vi "Meas_EIS_Spectra_Polar_v6 - temp.vi"(9 "output cluster":T1, 10 "testp":T2={"Start F"=1.0, "Stop F"=10000.0, "# Steps"=50, "Init Z Guess"=1.0, "Device #"=0, "Vdrive (V)"=0.1} caption="Test Parameters" {"Vdrive (V)" min=0.0001 max=10; "Device #" min=0 max=10 step=1; "Init Z Guess" format="%_5f"; "# Steps" min=1 max=1800 step=1; "Stop F" min=0.0010000000474974513 max=2000000.0 step=0.001 format="%#_3f"; "Start F" min=0.0010000000474974513 max=2000000.0 step=0.001 format="%#_3f"}, 11 "Output file refnum":refnum<file>) -> ()   [LabVIEW 2018]
uses:
  AC States cntrl.ctl
panel:
  out "Init Z Guess":sgl
  in  "Tab Control":enum32{"Outputs", "TakeData"}(tab)
  out "XY Graph":cluster{sgl, sgl}[](graph)
  out "IERange":i32
  out "IchRange":i32
  out "VchRange":i32
  out "Index no.":i32=1
  out "Zphz":dbl
  out "Zmod":dbl
  out "Zfreq":dbl
  in  "Control Mode":i32(ring)=1 items=["GstatMode", "PstatMode", "ZRAMode", "FRAMode"]
  out "Data Available":bool
  out "Status":enum16{"Ok", "Retry", "Error", "Done"}(ring)
  out "NumPoints":i32
  in  "Freqin":sgl=1000.0 format="%#_3g"
  out "event callback refnum":refnum<k27>
  out "Section":string
  out "ReadZ":refnum<k7>
  out "Pstat":refnum<k7>
  out "Device List":refnum<k7>
  out "Data Acquisition Complete":bool
  in  "GAMRYCOMLib.IGamryReadZ":refnum<k7>
  in  "GAMRYCOMLib.IGamryPstat":refnum<k7>
  in  "GAMRYCOMLib.IGamryDeviceList":refnum<k7>
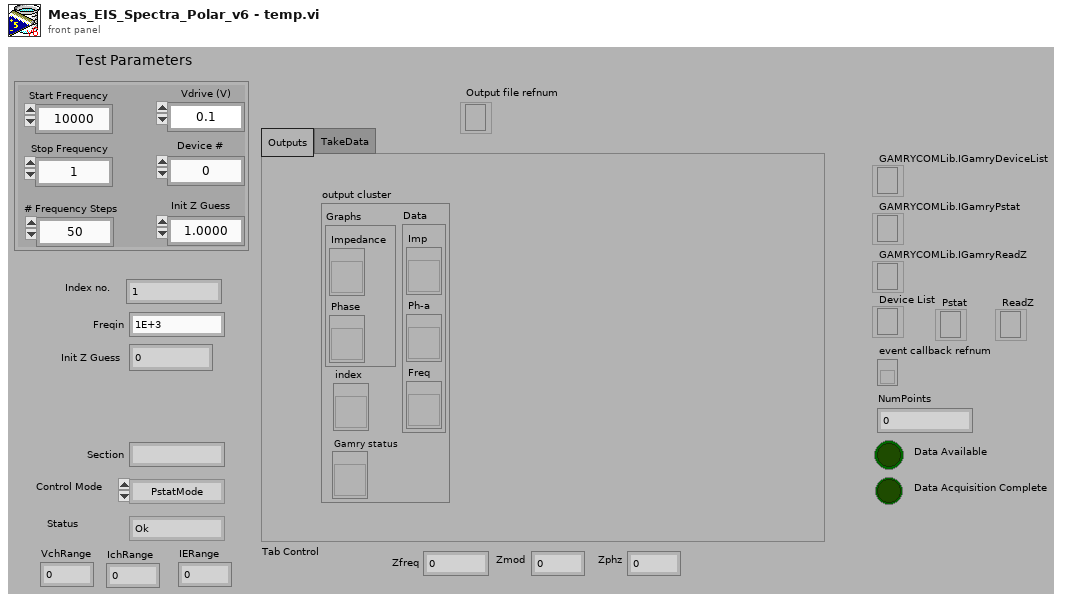
[diagram p1: front panel]
types:
  T1 = cluster{"Data":cluster{"Imp":refnum<vi>, "Ph-a":refnum<vi>, "Freq":refnum<vi>}, "Graphs":cluster{"Impedance":refnum<vi>, "Phase":refnum<vi>}, "index":refnum<vi>, "Gamry status":refnum<vi>}
  T2 = cluster{"Start F":dbl, "Stop F":dbl, "# Steps":u32, "Init Z Guess":sgl, "Device #":i16, "Vdrive (V)":sgl}
  T3 = typedef "AC States cntrl.ctl" = enum16{"Initialize Variables", "Initialize Pstat", "Initialize Dtaq", "Settings", "Frequency calc", "Set Cycle Limits", "Take Data", "Read Z Measure", "Cleanup", "Stop"}
  T4 = cluster{"Imp":refnum<vi>, "Ph-a":refnum<vi>, "Freq":refnum<vi>}
  T5 = cluster{"Impedance":refnum<vi>, "Phase":refnum<vi>}
  T6 = cluster{"Data Acquisition Complete":refnum<vi>, "Status":refnum<vi>}
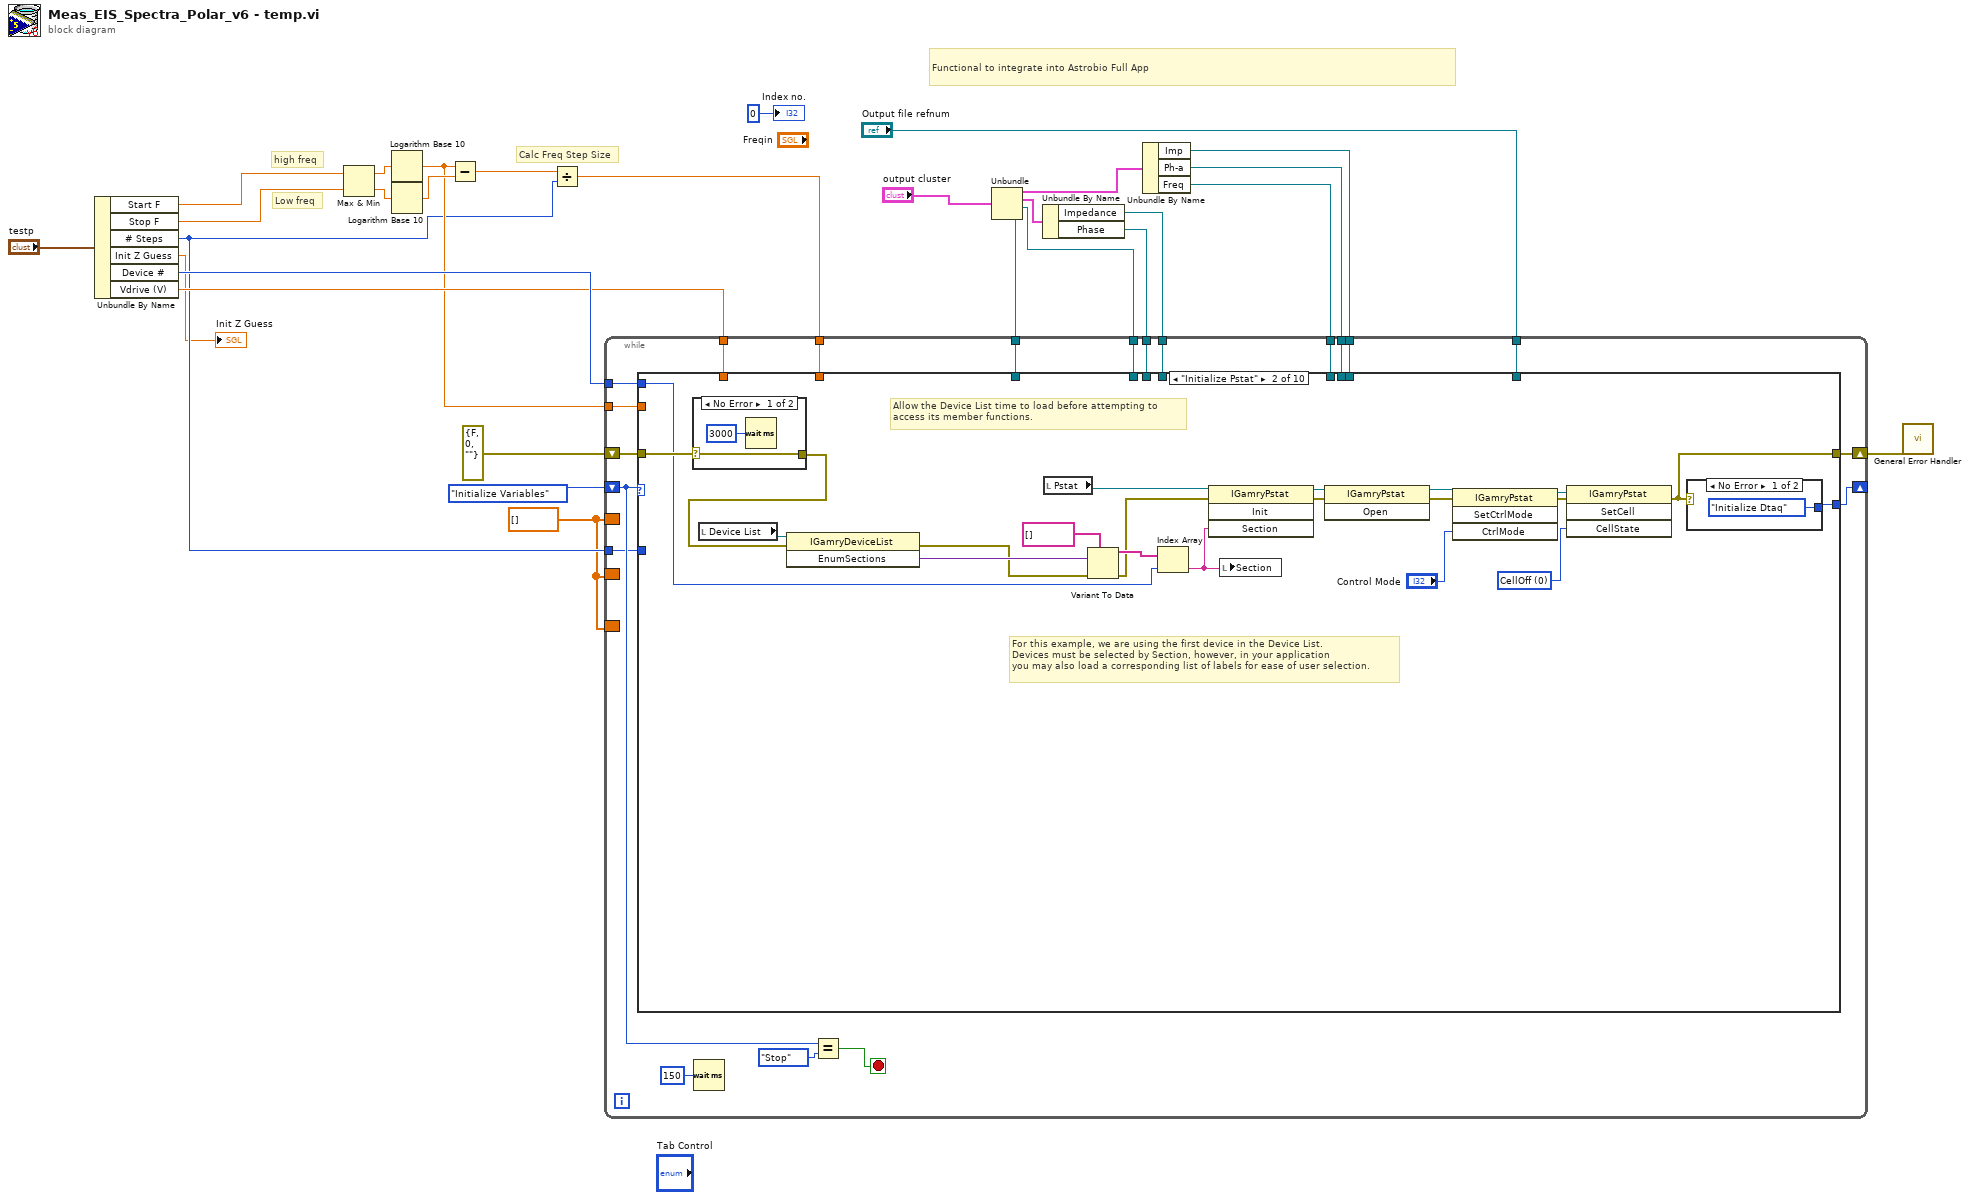
[diagram p0: block diagram]
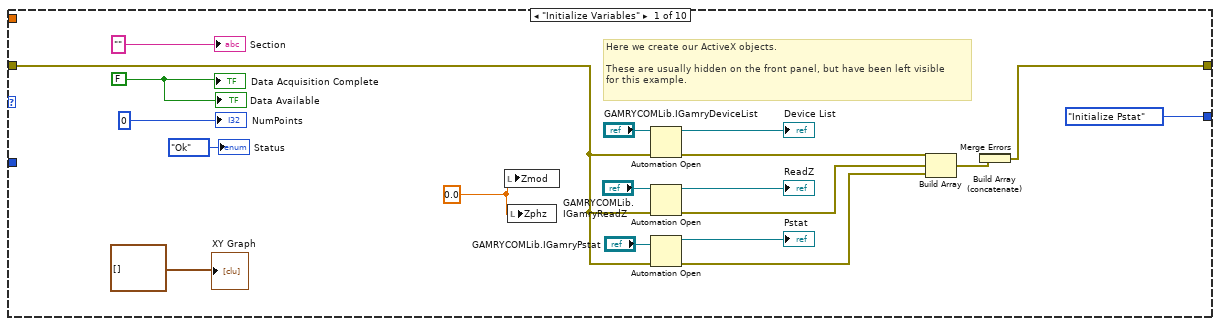
[diagram p2: hidden frame]
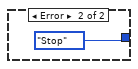
[diagram p4: hidden frame]
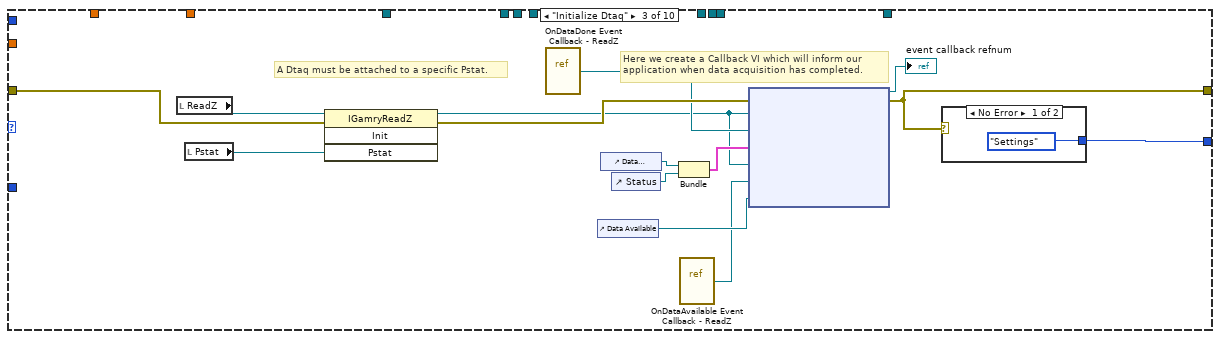
[diagram p5: hidden frame]
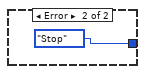
[diagram p6: hidden frame]
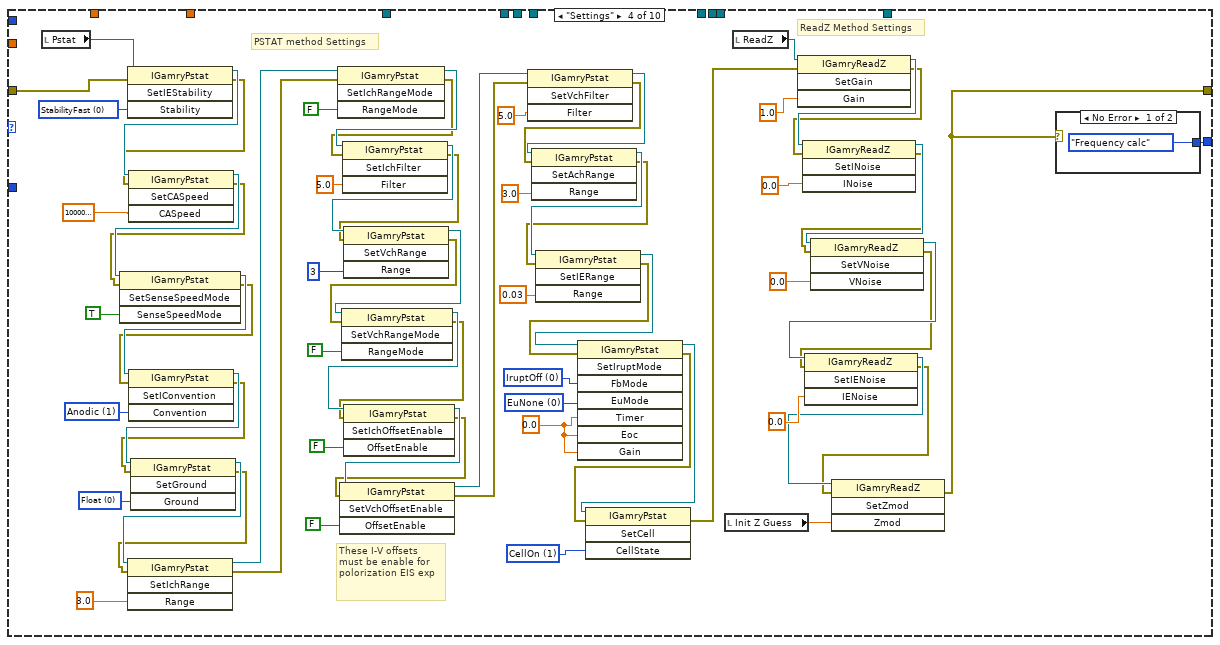
[diagram p7: hidden frame]
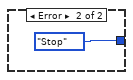
[diagram p8: hidden frame]
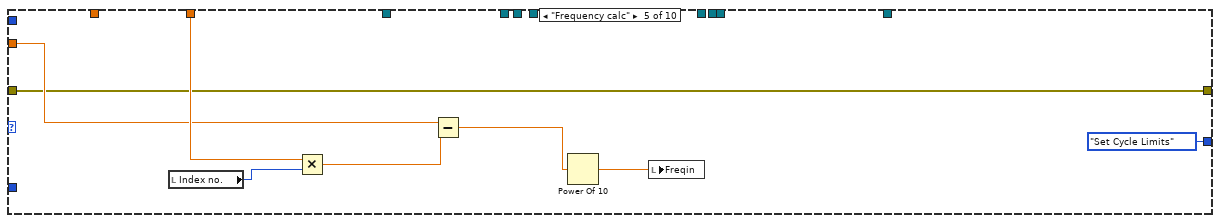
[diagram p9: hidden frame]
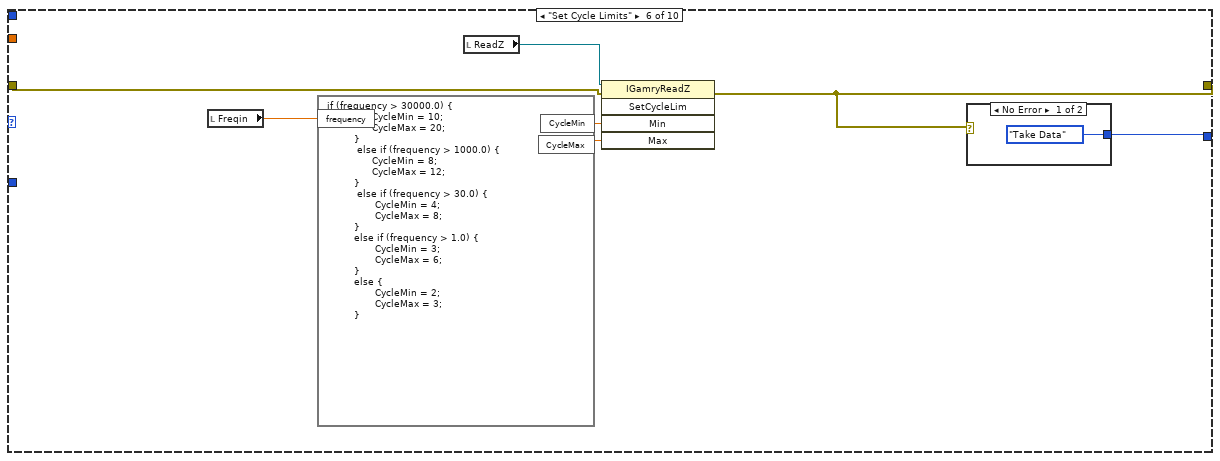
[diagram p10: hidden frame]
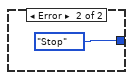
[diagram p11: hidden frame]
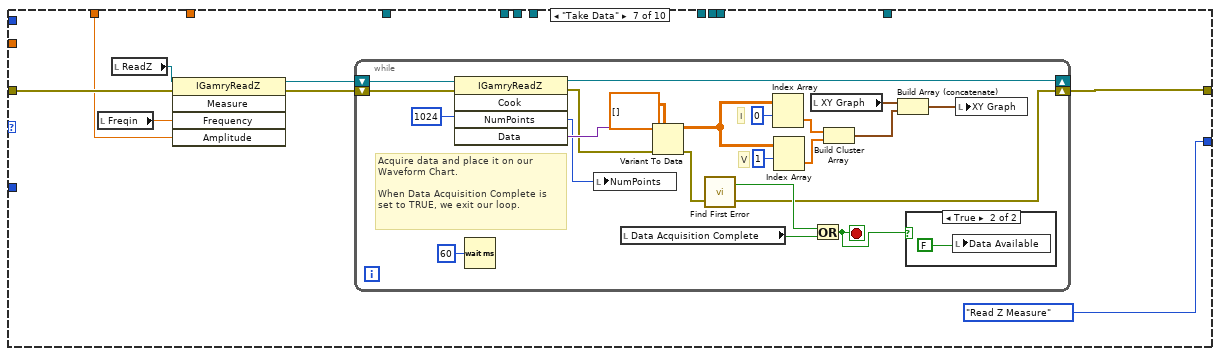
[diagram p12: hidden frame]
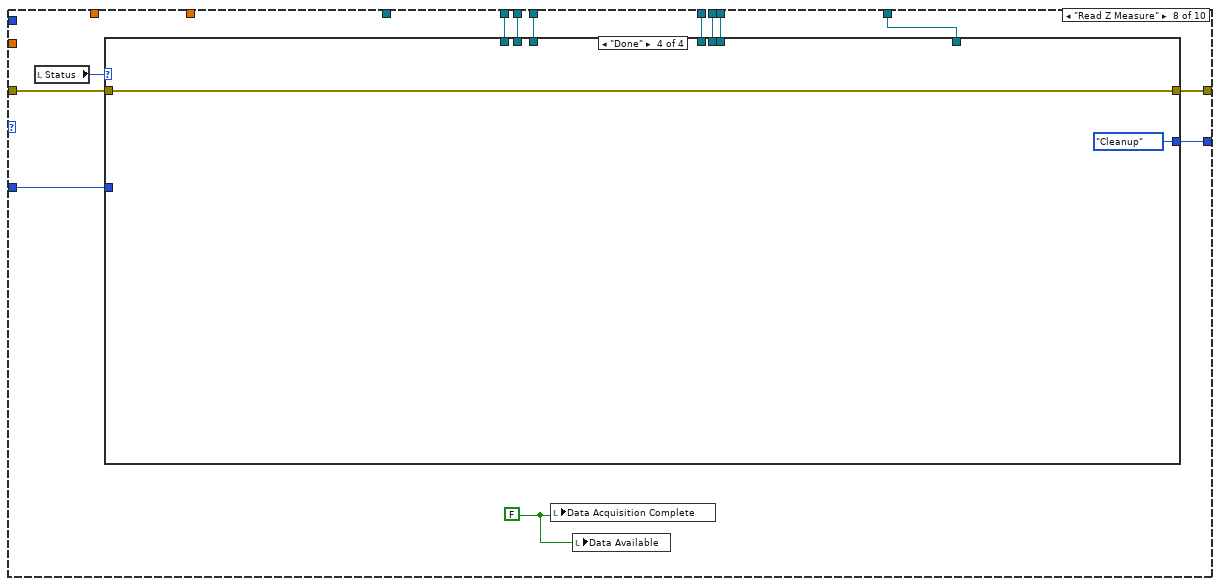
[diagram p14: hidden frame]
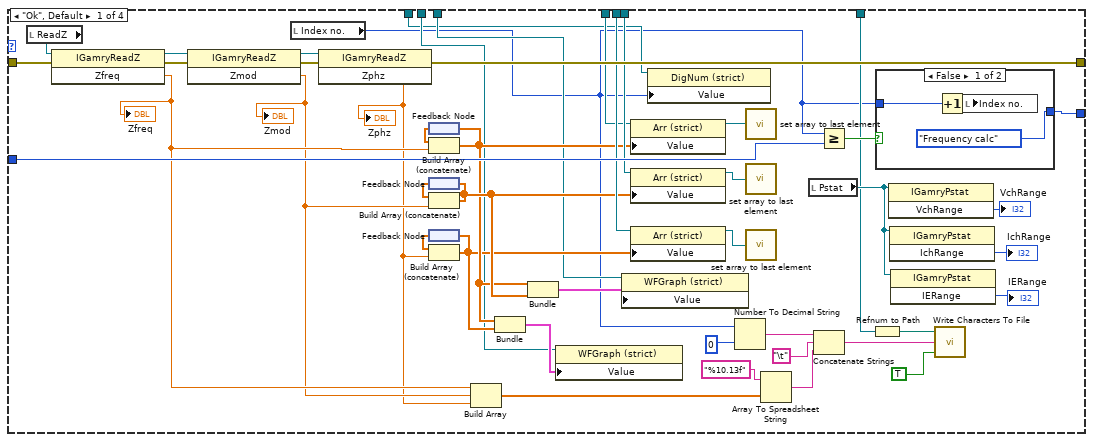
[diagram p15: hidden frame]
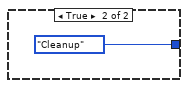
[diagram p16: hidden frame]
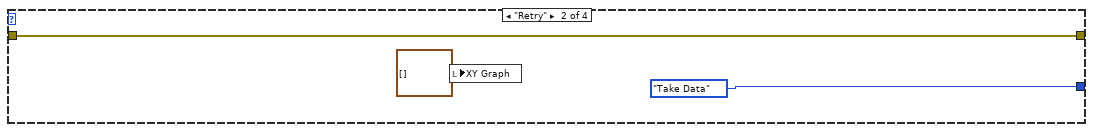
[diagram p17: hidden frame]
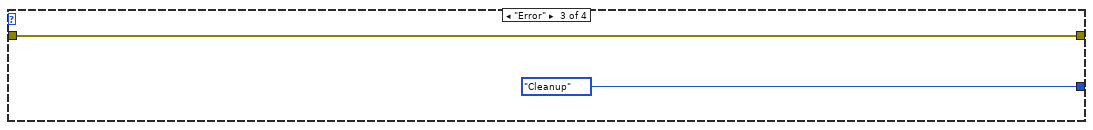
[diagram p18: hidden frame]
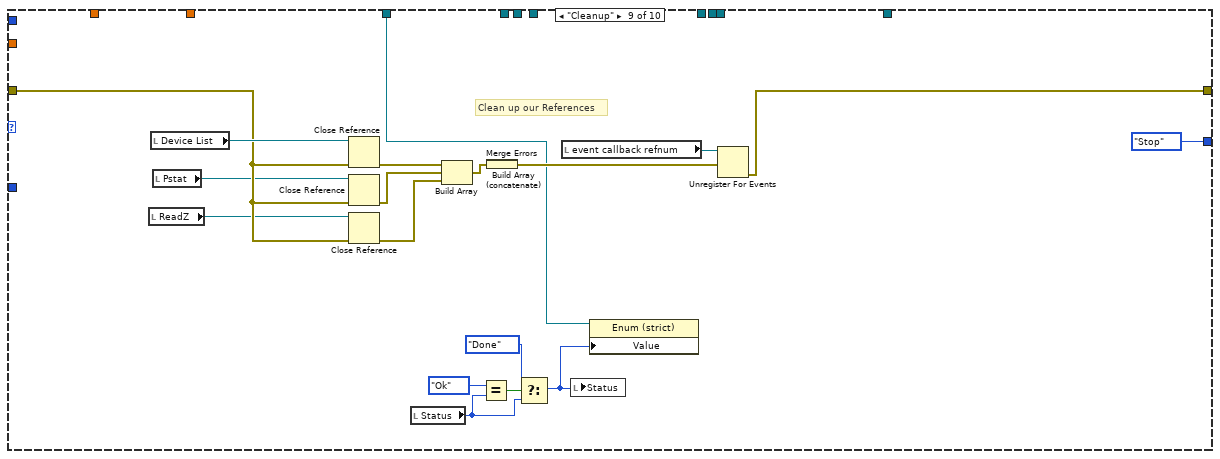
[diagram p19: hidden frame]
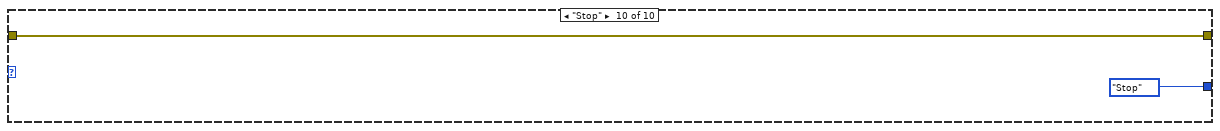
[diagram p20: hidden frame]
diagram:
  w3 = dbl[] []
  # "Functional to integrate into Astrobio Full App"
  # "Calc Freq Step Size"
  # "Low freq"
  # "high freq"
  n1 = Unbundle By Name("testp") -> ("Start F"=w19:dbl, "Stop F"=w18:dbl, "# Steps"=w14:u32, "Init Z Guess"=→"Init Z Guess":sgl, "Device #"=w25:i16, "Vdrive (V)"=w24:sgl)
  n2 = Max & Min(x=w19, y=w18) -> (max(x,y)=w22:dbl, min(x,y)=w23:dbl)
  n3 = Logarithm Base 10(1:w22) -> (0:w16:dbl)
  n4 = Logarithm Base 10(1:w23) -> (0:w20:dbl)
  n5 = Subtract(x=w16, y=w20) -> (x-y=w21:dbl)
  n6 = Divide(x=w21, y=w14) -> (x/y=w15:dbl)
  n7 = Unbundle("output cluster") -> ("Data"=w10:T4, "Graphs"=w6:T5, "index"=w1:refnum<vi>, "Gamry status"=w2:refnum<vi>)
  n8 = Unbundle By Name(w6) -> ("Impedance"=w5:refnum<vi>, "Phase"=w4:refnum<vi>)
  n9 = Unbundle By Name(w10) -> ("Imp"=w9:refnum<vi>, "Ph-a"=w8:refnum<vi>, "Freq"=w7:refnum<vi>)
  n10 = while {
    shift-right: [w46] -> _
    shift-left: AC_States_cntrl."Initialize Variables" ("DC Demo States") -> [w47]
    shift-right: [w44] -> w28
    shift-left: errorcluster {"status"=FALSE, "code"=0, "source"=""} ("error in (no error)") -> [w45]
    tunnel: w24 -> [w42]
    tunnel: w25 -> [w41]
    tunnel: w14 -> [w40]
    tunnel: w16 -> [w39]
    tunnel: w15 -> [w38]
    tunnel: "Output file refnum" -> [w37]
    border: w3 -> [_]
    border: w3 -> [_]
    border: w3 -> [_]
    tunnel: w9 -> [w36]
    tunnel: w8 -> [w35]
    tunnel: w7 -> [w34]
    tunnel: w5 -> [w33]
    tunnel: w4 -> [w32]
    tunnel: w1 -> [w31]
    tunnel: w2 -> [w30]
    stop <- w48 stop-if-true
    n11 = case shown="\"Initialize Pstat\"" w47 {
      tunnel: [AC_States_cntrl."Initialize Pstat" ("DC Demo States") w86 w108 w180 AC_States_cntrl."Set Cycle Limits" ("DC Demo States") w198 AC_States_cntrl."Read Z Measure" ("DC Demo States") w243 AC_States_cntrl."Stop" ("DC Demo States") AC_States_cntrl."Stop" ("DC Demo States")] -> w46
      tunnel: w45 -> [w58 w77 w106 w161 w184 w197 w207 w242 w317 w320]
      tunnel: [w59 w70 w105 w179 w184 w192 w206 w241 w308 w320] -> w44
      tunnel: w42 -> [_ _ _ _ _ _ w202 _ _ _]
      tunnel: w41 -> [_ w74 _ _ _ _ _ _ _ _]
      tunnel: w40 -> [_ _ _ _ _ _ _ w240 _ _]
      tunnel: w39 -> [_ _ _ _ w189 _ _ _ _ _]
      tunnel: w38 -> [_ _ _ _ w190 _ _ _ _ _]
      tunnel: w37 -> [_ _ _ _ _ _ _ w239 _ _]
      tunnel: w36 -> [_ _ _ _ _ _ _ w237 _ _]
      tunnel: w35 -> [_ _ _ _ _ _ _ w236 _ _]
      tunnel: w34 -> [_ _ _ _ _ _ _ w235 _ _]
      tunnel: w33 -> [_ _ _ _ _ _ _ w234 _ _]
      tunnel: w32 -> [_ _ _ _ _ _ _ w233 _ _]
      tunnel: w31 -> [_ _ _ _ _ _ _ w232 _ _]
      tunnel: w30 -> [_ _ _ _ _ _ _ _ w305 _]
      frame "Initialize Variables" {
        w52 = sgl 0.0 ("Zreal")
        w54 = FALSE
        # "Here we create our ActiveX objects.\n\nThese are usually hidden on the front panel, but have been left visible\nfor this example."
        n12 = local write "Zmod"(w52) -> ()
        n13 = local write "Zphz"(w52) -> ()
        n14 = Automation Open(error in (no error)=w58, Automation Refnum="GAMRYCOMLib.IGamryDeviceList") -> (Automation Refnum=→"Device List":refnum<k7>, error out=w61:errorcluster)  [unwired: 2 in]
        n15 = Automation Open(error in (no error)=w58, Automation Refnum="GAMRYCOMLib.IGamryReadZ") -> (Automation Refnum=→"ReadZ":refnum<k7>, error out=w56:errorcluster)  [unwired: 2 in]
        n16 = Automation Open(error in (no error)=w58, Automation Refnum="GAMRYCOMLib.IGamryPstat") -> (Automation Refnum=→"Pstat":refnum<k7>, error out=w57:errorcluster)  [unwired: 2 in]
        n17 = Build Array(w61, w56, w57) -> (w60:errorcluster[])
        n18 = Build Array (concatenate)(w60) -> (w53:errorcluster[])
        n19 = Merge Errors(w53) -> (w59:errorcluster)
        "Data Acquisition Complete" <- w54
        "Section" <- "" ("Section")
        "NumPoints" <- 0 ("NumPoints")
        "Data Available" <- w54
        "XY Graph" <- cluster{sgl, sgl}[] [] ("appended array")
        "Status" <- enum16{"Ok", "Retry", "Error", "Done"}."Ok" ("Status")
      }
      frame "Initialize Pstat" {
        w73 = 0 items=["CellOff", "CellOn"] ("CellState")
        # "For this example, we are using the first device in the Device List.\nDevices must be selected by Section, however, in your application\nyou may also load a corresponding list of labels for ease of user selection."
        # "Allow the Device List time to load before attempting to \naccess its member functions."
        n20 = case shown="No Error" w77 {
          selector: w77 -> [w91 w93]
          tunnel: [w91 w93] -> w76
          frame No Error {
            n21 = Wait (ms)(milliseconds to wait=u32 3000) -> ()  [unwired: 1 out]
          }
          frame Error {
          }
        }
        n22 = local read "Device List"() -> (w81:refnum<k7>)
        n23 = invoke class="IGamryDeviceList" method="EnumSections"(reference=w81, error in=w76) -> (error out=w79:errorcluster, "EnumSections"=w80:variant)  [unwired: 1 in, 1 out]
        n24 = local read "Pstat"() -> (w83:refnum<k7>)
        n25 = Variant To Data(error in=w79, type=string[] [], Variant=w80) -> (data=w85:string[], error out=w78:errorcluster)
        n26 = Index Array(array=w85, index=w74) -> (element=w82:string)
        n27 = invoke class="IGamryPstat" method="Init"(reference=w83, error in=w78, "Section"=w82) -> (reference out=w90:refnum<k7>, error out=w89:errorcluster)  [unwired: 1 in, 2 out]
        n28 = local write "Section"(w82) -> ()
        n29 = invoke class="IGamryPstat" method="Open"(reference=w90, error in=w89) -> (reference out=w87:refnum<k7>, error out=w88:errorcluster)  [unwired: 1 in, 1 out]
        n30 = invoke class="IGamryPstat" method="SetCtrlMode"(reference=w87, error in=w88, "CtrlMode"="Control Mode") -> (reference out=w72:refnum<k7>, error out=w71:errorcluster)  [unwired: 1 in, 2 out]
        n31 = invoke class="IGamryPstat" method="SetCell"(reference=w72, error in=w71, "CellState"=w73) -> (error out=w70:errorcluster)  [unwired: 1 in, 3 out]
        n32 = case shown="No Error" w70 {
          tunnel: [AC_States_cntrl."Initialize Dtaq" ("DC Demo States") AC_States_cntrl."Stop" ("DC Demo States")] -> w86
          frame No Error {
          }
          frame Error {
          }
        }
      }
      frame "Initialize Dtaq" {
        # "A Dtaq must be attached to a specific Pstat."
        # "Here we create a Callback VI which will inform our\napplication when data acquisition has completed."
        n33 = local read "ReadZ"() -> (w107:refnum<k7>)
        n34 = local read "Pstat"() -> (w109:refnum<k7>)
        n35 = invoke class="IGamryReadZ" method="Init"(reference=w107, error in=w106, "Pstat"=w109) -> (reference out=w97:refnum<k7>, error out=w103:errorcluster)  [unwired: 1 in, 2 out]
        n36 = vi-ref "OnDataDone Event Callback - ReadZ.vi"() -> ("vi reference"=w99:refnum<vi>)
        n37 = control-ref of="Data Available"() -> (w98:refnum<vi>)
        n38 = control-ref of="Data Acquisition Complete"() -> (w102:refnum<vi>)
        n39 = control-ref of="Status"() -> (w101:refnum<vi>)
        n40 = Bundle("Data Acquisition Complete"=w102, "Status"=w101) -> (w100:T6)  [unwired: 1 in]
        n41 = vi-ref "OnDataAvailable Event Callback - ReadZ.vi"() -> ("vi reference"=w96:refnum<vi>)
        n42 = node(w103, w97, w99, w100, w97, w96, w98) -> (→"event callback refnum":refnum<k27>, w105:errorcluster)  [unwired: 1 in]
        n43 = case shown="No Error" w105 {
          tunnel: [AC_States_cntrl."Settings" ("DC Demo States") AC_States_cntrl."Stop" ("DC Demo States")] -> w108
          frame No Error {
          }
          frame Error {
          }
        }
      }
      frame "Settings" {
        w115 = sgl 0.0 ("Timer")
        w116 = 0 items=["EuNone", "EuExtrap", "EuAverage"] ("EuMode")
        w117 = 0 items=["IruptOff", "IruptNorm", "IruptClfg"] ("FbMode")
        w150 = 0 items=["Float", "Earth"] ("Ground")
        w153 = 1 items=["Cathodic", "Anodic"] ("Convention")
        w160 = 0 items=["StabilityFast", "StabilityMedFast", "StabilityNorm", "StabilitySlow"] ("Stability")
        w181 = 1 items=["CellOff", "CellOn"] ("CellState")
        # "ReadZ Method Settings"
        # "These I-V offsets must be enable for polorization EIS exp"
        # "PSTAT method Settings"
        n44 = local read "Pstat"() -> (w162:refnum<k7>)
        n45 = invoke class="IGamryPstat" method="SetIEStability"(reference=w162, error in=w161, "Stability"=w160) -> (reference out=w159:refnum<k7>, error out=w158:errorcluster)  [unwired: 1 in, 2 out]
        n46 = invoke class="IGamryPstat" method="SetCASpeed"(reference=w159, error in=w158, "CASpeed"=1000000.0) -> (reference out=w155:refnum<k7>, error out=w154:errorcluster)  [unwired: 1 in, 2 out]
        n47 = invoke class="IGamryPstat" method="SetSenseSpeedMode"(reference=w155, error in=w154, "SenseSpeedMode"=TRUE) -> (reference out=w152:refnum<k7>, error out=w151:errorcluster)  [unwired: 1 in, 2 out]
        n48 = invoke class="IGamryPstat" method="SetIConvention"(reference=w152, error in=w151, "Convention"=w153) -> (reference out=w149:refnum<k7>, error out=w148:errorcluster)  [unwired: 1 in, 2 out]
        n49 = invoke class="IGamryPstat" method="SetGround"(reference=w149, error in=w148, "Ground"=w150) -> (reference out=w146:refnum<k7>, error out=w145:errorcluster)  [unwired: 1 in, 2 out]
        n50 = invoke class="IGamryPstat" method="SetIchRange"(reference=w146, error in=w145, "Range"=3.0) -> (reference out=w144:refnum<k7>, error out=w143:errorcluster)  [unwired: 1 in, 2 out]
        n51 = invoke class="IGamryPstat" method="SetIchRangeMode"(reference=w144, error in=w143, "RangeMode"=FALSE) -> (reference out=w140:refnum<k7>, error out=w139:errorcluster)  [unwired: 1 in, 2 out]
        n52 = invoke class="IGamryPstat" method="SetIchFilter"(reference=w140, error in=w139, "Filter"=5.0) -> (reference out=w138:refnum<k7>, error out=w137:errorcluster)  [unwired: 1 in, 2 out]
        n53 = invoke class="IGamryPstat" method="SetVchRange"(reference=w138, error in=w137, "Range"=3) -> (reference out=w135:refnum<k7>, error out=w134:errorcluster)  [unwired: 1 in, 2 out]
        n54 = invoke class="IGamryPstat" method="SetVchRangeMode"(reference=w135, error in=w134, "RangeMode"=FALSE) -> (reference out=w133:refnum<k7>, error out=w132:errorcluster)  [unwired: 1 in, 2 out]
        n55 = invoke class="IGamryPstat" method="SetIchOffsetEnable"(reference=w133, error in=w132, "OffsetEnable"=FALSE) -> (reference out=w129:refnum<k7>, error out=w128:errorcluster)  [unwired: 1 in, 2 out]
        n56 = invoke class="IGamryPstat" method="SetVchOffsetEnable"(reference=w129, error in=w128, "OffsetEnable"=FALSE) -> (reference out=w127:refnum<k7>, error out=w126:errorcluster)  [unwired: 1 in, 2 out]
        n57 = invoke class="IGamryPstat" method="SetVchFilter"(reference=w127, error in=w126, "Filter"=5.0) -> (reference out=w123:refnum<k7>, error out=w122:errorcluster)  [unwired: 1 in, 2 out]
        n58 = invoke class="IGamryPstat" method="SetAchRange"(reference=w123, error in=w122, "Range"=3.0) -> (reference out=w121:refnum<k7>, error out=w120:errorcluster)  [unwired: 1 in, 2 out]
        n59 = invoke class="IGamryPstat" method="SetIERange"(reference=w121, error in=w120, "Range"=0.03) -> (reference out=w119:refnum<k7>, error out=w118:errorcluster)  [unwired: 1 in, 2 out]
        n60 = invoke class="IGamryPstat" method="SetIruptMode"(reference=w119, error in=w118, "FbMode"=w117, "EuMode"=w116, "Timer"=w115, "Eoc"=w115, "Gain"=w115) -> (reference out=w114:refnum<k7>, error out=w113:errorcluster)  [unwired: 1 in, 6 out]
        n61 = invoke class="IGamryPstat" method="SetCell"(reference=w114, error in=w113, "CellState"=w181) -> (error out=w176:errorcluster)  [unwired: 1 in, 3 out]
        n62 = local read "Init Z Guess"() -> (w112:sgl)
        n63 = local read "ReadZ"() -> (w177:refnum<k7>)
        n64 = invoke class="IGamryReadZ" method="SetGain"(reference=w177, error in=w176, "Gain"=sgl 1.0 ("Zmod")) -> (reference out=w174:refnum<k7>, error out=w173:errorcluster)  [unwired: 1 in, 2 out]
        n65 = invoke class="IGamryReadZ" method="SetINoise"(reference=w174, error in=w173, "INoise"=sgl 0.0 ("Zmod")) -> (reference out=w171:refnum<k7>, error out=w170:errorcluster)  [unwired: 1 in, 2 out]
        n66 = invoke class="IGamryReadZ" method="SetVNoise"(reference=w171, error in=w170, "VNoise"=sgl 0.0 ("Zmod")) -> (reference out=w168:refnum<k7>, error out=w167:errorcluster)  [unwired: 1 in, 2 out]
        n67 = invoke class="IGamryReadZ" method="SetIENoise"(reference=w168, error in=w167, "IENoise"=sgl 0.0 ("Zmod")) -> (reference out=w166:refnum<k7>, error out=w165:errorcluster)  [unwired: 1 in, 2 out]
        n68 = invoke class="IGamryReadZ" method="SetZmod"(reference=w166, error in=w165, "Zmod"=w112) -> (error out=w179:errorcluster)  [unwired: 1 in, 3 out]
        n69 = case shown="No Error" w179 {
          tunnel: [AC_States_cntrl."Frequency calc" ("DC Demo States") AC_States_cntrl."Stop" ("DC Demo States")] -> w180
          frame No Error {
          }
          frame Error {
          }
        }
      }
      frame "Frequency calc" {
        n70 = local read "Index no."() -> (w191:i32)
        n71 = Multiply(x=w190, y=w191) -> (x*y=w188:dbl)
        n72 = Subtract(x=w189, y=w188) -> (x-y=w187:dbl)
        n73 = Power Of 10(x=w187) -> (10^x=w186:dbl)
        n74 = local write "Freqin"(w186) -> ()
      }
      frame "Set Cycle Limits" {
        n75 = local read "Freqin"() -> (w195:sgl)
        n76 = formula code="if (frequency > 30000.0) {\n               CycleMin = 10;\n               CycleMax = 20;\n         }\n          else if (frequency > 1000.0) {\n               CycleMin = 8;\n               CycleMax = 12;\n         }\n          else if (frequency > 30.0) {\n                CycleMin = 4;\n                CycleMax = 8;\n         }\n         else if (frequency > 1.0) {\n                CycleMin = 3;\n                CycleMax = 6;\n         }\n         else {\n                CycleMin = 2;\n                CycleMax = 3;\n         }"("frequency"=w195) -> ("CycleMin"=w194:dbl, "CycleMax"=w193:dbl)
        n77 = local read "ReadZ"() -> (w196:refnum<k7>)
        n78 = invoke class="IGamryReadZ" method="SetCycleLim"(reference=w196, error in=w197, "Min"=w194, "Max"=w193) -> (error out=w192:errorcluster)  [unwired: 1 in, 4 out]
        n79 = case shown="No Error" w192 {
          tunnel: [AC_States_cntrl."Take Data" ("DC Demo States") AC_States_cntrl."Stop" ("DC Demo States")] -> w198
          frame No Error {
          }
          frame Error {
          }
        }
      }
      frame "Take Data" {
        n80 = local read "Freqin"() -> (w201:sgl)
        n81 = local read "ReadZ"() -> (w205:refnum<k7>)
        n82 = invoke class="IGamryReadZ" method="Measure"(reference=w205, error in=w207, "Frequency"=w201, "Amplitude"=w202) -> (reference out=w204:refnum<k7>, error out=w203:errorcluster)  [unwired: 1 in, 3 out]
        n83 = while {
          shift-right: [w221] -> w206
          shift-left: w203 -> [w229]
          shift-right: [w220] -> _
          shift-left: w204 -> [w230]
          stop <- w209 stop-if-true
          # "V"
          # "I"
          # "Acquire data and place it on our\nWaveform Chart.\n\nWhen Data Acquisition Complete is\nset to TRUE, we exit our loop."
          n84 = invoke class="IGamryReadZ" method="Cook"(reference=w230, error in=w229, "NumPoints"=1024) -> (reference out=w220:refnum<k7>, error out=w225:errorcluster, "NumPoints"=w215:i32, "Data"=w226:variant)  [unwired: 2 in, 1 out]
          n85 = Wait (ms)(milliseconds to wait=u32 60) -> ()  [unwired: 1 out]
          n86 = local write "NumPoints"(w215) -> ()
          n87 = local read "Data Acquisition Complete"() -> (w222:bool)
          n88 = Variant To Data(error in=w225, type=sgl[][] [], Variant=w226) -> (data=w216:sgl[][], error out=w224:errorcluster)
          n89 = call <vilib>:"Find First Error.vi"("error in (no error)"=w224) -> ("error out"=w221:errorcluster, "error?"=w223:bool)  [unwired: 3 in]
          n90 = Index Array(array=w216, index (row)=0) -> (element=w214:sgl[])  [unwired: 1 in]
          n91 = Index Array(array=w216, index (row)=1) -> (element=w213:sgl[])  [unwired: 1 in]
          n92 = local read "XY Graph"() -> (w212:cluster{sgl, sgl}[])
          n93 = Or(x=w223, y=w222) -> (x .or. y?=w209:bool)
          n94 = Build Cluster Array(w214, w213) -> (w211:cluster{sgl, sgl}[])
          n95 = Build Array (concatenate)(w212, w211) -> (w210:cluster{sgl, sgl}[])
          n96 = case shown="True" w209 {
            frame False {
            }
            frame True {
              n97 = local write "Data Available"(FALSE) -> ()
            }
          }
          n98 = local write "XY Graph"(w210) -> ()
        }
      }
      frame "Read Z Measure" {
        w238 = FALSE
        n99 = local read "Status"() -> (w244:enum16{"Ok", "Retry", "Error", "Done"})
        n100 = case shown="\"Done\"" w244 {
          tunnel: [w276 AC_States_cntrl."Take Data" ("DC Demo States") AC_States_cntrl."Cleanup" ("DC Demo States") AC_States_cntrl."Cleanup" ("DC Demo States")] -> w243
          tunnel: w242 -> [w286 w295 w297 w300]
          tunnel: [w287 w295 w297 w300] -> w241
          tunnel: w240 -> [w278 _ _ _]
          tunnel: w239 -> [w267 _ _ _]
          tunnel: w237 -> [w259 _ _ _]
          tunnel: w236 -> [w258 _ _ _]
          tunnel: w235 -> [w257 _ _ _]
          tunnel: w234 -> [w251 _ _ _]
          tunnel: w233 -> [w250 _ _ _]
          tunnel: w232 -> [w249 _ _ _]
          frame "Ok", Default {
            n101 = local read "ReadZ"() -> (w283:refnum<k7>)
            n102 = invoke class="IGamryReadZ" method="Zfreq"(reference=w283, error in=w286) -> (reference out=w284:refnum<k7>, error out=w285:errorcluster, "Zfreq"=w263:sgl)  [unwired: 1 in]
            "Zfreq" <- w263
            n103 = invoke class="IGamryReadZ" method="Zmod"(reference=w284, error in=w285) -> (reference out=w288:refnum<k7>, error out=w289:errorcluster, "Zmod"=w262:sgl)  [unwired: 1 in]
            "Zmod" <- w262
            n104 = local read "Index no."() -> (w248:i32)
            n105 = invoke class="IGamryReadZ" method="Zphz"(reference=w288, error in=w289) -> (error out=w287:errorcluster, "Zphz"=w260:sgl)  [unwired: 1 in, 1 out]
            "Zphz" <- w260
            n106 = feedback #1() -> (w246:dbl[])
            n107 = Build Array (concatenate)(w246, w263) -> (w254:dbl[])
            n108 = feedback-in #1(w254) -> ()
            n109 = feedback #2() -> (w261:dbl[])
            n110 = Build Array (concatenate)(w261, w262) -> (w255:dbl[])
            n111 = feedback-in #2(w255) -> ()
            n112 = feedback #3() -> (w247:dbl[])
            n113 = Build Array (concatenate)(w247, w260) -> (w253:dbl[])
            n114 = feedback-in #3(w253) -> ()
            n115 = Build Array(w263, w262, w260) -> (w273:sgl[])
            n116 = Bundle(w254, w253) -> (w252:cluster{dbl[], dbl[]})  [unwired: 1 in]
            n117 = Bundle(w254, w255) -> (w256:cluster{dbl[], dbl[]})  [unwired: 1 in]
            n118 = property class="WFGraph (strict)"(reference=w250, "Value"=w252) -> ()  [unwired: 1 in, 2 out]
            n119 = property class="WFGraph (strict)"(reference=w251, "Value"=w256) -> ()  [unwired: 1 in, 2 out]
            n120 = property class="Arr (strict)"(reference=w257, "Value"=w254) -> (reference out=w266:refnum<vi>)  [unwired: 1 in, 1 out]
            n121 = property class="Arr (strict)"(reference=w259, "Value"=w255) -> (reference out=w265:refnum<vi>)  [unwired: 1 in, 1 out]
            n122 = property class="Arr (strict)"(reference=w258, "Value"=w253) -> (reference out=w264:refnum<vi>)  [unwired: 1 in, 1 out]
            n123 = property class="DigNum (strict)"(reference=w249, "Value"=w248) -> ()  [unwired: 1 in, 2 out]
            n124 = Number To Decimal String(number=w248, width (-)=i16 0) -> (decimal integer string=w270:string)
            n125 = call "set array to last element.vi"("Arr Refnum"=w266) -> ()
            n126 = call "set array to last element.vi"("Arr Refnum"=w265) -> ()
            n127 = call "set array to last element.vi"("Arr Refnum"=w264) -> ()
            n128 = Array To Spreadsheet String(array=w273, 3:"%10.13f") -> (spreadsheet string=w269:string)  [unwired: 1 in]
            n129 = local read "Pstat"() -> (w282:refnum<k7>)
            n130 = Concatenate Strings(w270, "\t", w269) -> (w268:string)
            n131 = Greater Or Equal?(x=w248, y=w278) -> (x >= y?=w277:bool)
            n132 = Refnum to Path(1:w267) -> (0:w245:path)
            n133 = case shown="False" w277 {
              tunnel: [AC_States_cntrl."Frequency calc" ("DC Demo States") AC_States_cntrl."Cleanup" ("DC Demo States")] -> w276
              tunnel: w248 -> [w290 _]
              frame False {
                n134 = Increment(x=w290) -> (x+1=w291:i32)
                n135 = local write "Index no."(w291) -> ()
              }
              frame True {
              }
            }
            n136 = invoke class="IGamryPstat" method="VchRange"(reference=w282) -> ("VchRange"=→"VchRange":i32)  [unwired: 2 in, 2 out]
            n137 = invoke class="IGamryPstat" method="IchRange"(reference=w282) -> ("IchRange"=→"IchRange":i32)  [unwired: 2 in, 2 out]
            n138 = invoke class="IGamryPstat" method="IERange"(reference=w282) -> ("IERange"=→"IERange":i32)  [unwired: 2 in, 2 out]
            n139 = call <vilib>:"Write Characters To File.vi"("append to file? (new file:F)"=TRUE, "character string"=w268, "file path (dialog if empty)"=w245) -> ()  [unwired: 2 in, 1 out]
          }
          frame "Retry" {
            n140 = local write "XY Graph"(cluster{sgl, sgl}[] [] ("appended array")) -> ()
          }
          frame "Error" {
          }
          frame "Done" {
          }
        }
        n141 = local write "Data Acquisition Complete"(w238) -> ()
        n142 = local write "Data Available"(w238) -> ()
      }
      frame "Cleanup" {
        # "Clean up our References"
        n143 = local read "ReadZ"() -> (w315:refnum<k7>)
        n144 = local read "Device List"() -> (w318:refnum<k7>)
        n145 = local read "Pstat"() -> (w316:refnum<k7>)
        n146 = Close Reference(reference=w318, error in (no error)=w317) -> (error out=w314:errorcluster)
        n147 = Close Reference(reference=w316, error in (no error)=w317) -> (error out=w313:errorcluster)
        n148 = Close Reference(reference=w315, error in (no error)=w317) -> (error out=w312:errorcluster)
        n149 = local read "Status"() -> (w301:enum16{"Ok", "Retry", "Error", "Done"})
        n150 = Build Array(w314, w313, w312) -> (w311:errorcluster[])
        n151 = Equal?(x=enum16{"Ok", "Retry", "Error", "Done"}."Ok", y=w301) -> (x = y?=w306:bool)
        n152 = Build Array (concatenate)(w311) -> (w307:errorcluster[])
        n153 = Merge Errors(w307) -> (w309:errorcluster)
        n154 = Select(t=enum16{"Ok", "Retry", "Error", "Done"}."Done", s=w306, f=w301) -> (s? t:f=w304:enum16{"Ok", "Retry", "Error", "Done"})
        n155 = local read "event callback refnum"() -> (w310:refnum<k27>)
        n156 = local write "Status"(w304) -> ()
        n157 = property class="Enum (strict)"(reference=w305, "Value"=w304) -> ()  [unwired: 1 in, 2 out]
        n158 = Unregister For Events(event registration refnum=w310, error in=w309) -> (error out=w308:errorcluster)
      }
      frame "Stop" {
      }
    }
    n159 = Wait (ms)(milliseconds to wait=u32 150) -> ()  [unwired: 1 out]
    n160 = Equal?(x=w47, y=AC_States_cntrl."Stop" ("DC Demo States")) -> (x = y?=w48:bool)
  }
  n161 = call <vilib>:"General Error Handler.vi"("error in (no error)"=w28) -> ()  [unwired: 10 in, 5 out]
  "Index no." <- 0 ("Index no.")
